vi "LVClass_Image get saturation.vi"(0 "Image in":refnum<class "Image.lvclass">, 7 "Pixels to Average":u32, 11 "error in (no error)":errorcluster) -> (4 "Image out":refnum<class "Image.lvclass">, 10 "Fill Percent":sgl, 15 "error out":errorcluster)   [LabVIEW 2020, in "Image.lvclass"]
doc: "Image statistics computation.\n\n--------------------------------------------------------------------------------\n\n<B>ImageIn </B> : Image object.\n<B>ImageOut </B> : Image object.\n<B>nb_extreme_pixels </B> : Number of pixels to average for min or max computation.\n<B>min </B> : Average of the nb_extreme_pixels greatest elements.\n<B>max </B> : Average of the nb_extreme_pixels smallest elements.\n<B>fill_percentage </B> : Percentage of saturated pixels.\n<B>ErrorIn </B> : Error\n<B>ErrorOut </B> : Error\n\n--------------------------------------------------------------------------------"
uses:
  Image.lvclass
  Image.lvclass/Image.ctl
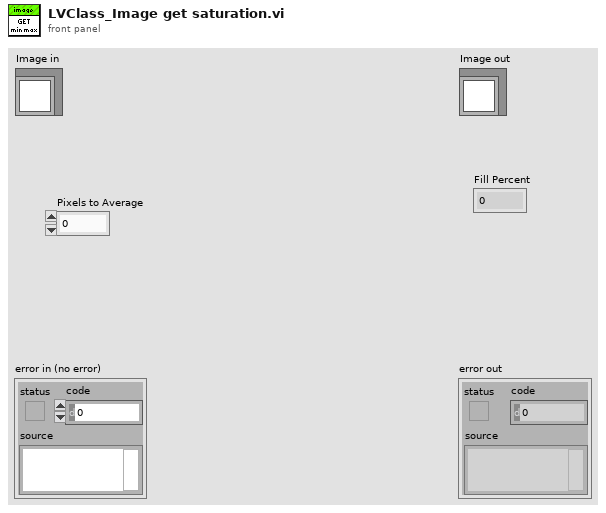
[diagram p1: front panel]
types:
  T1 = typedef "ClassID.ctl" = i64
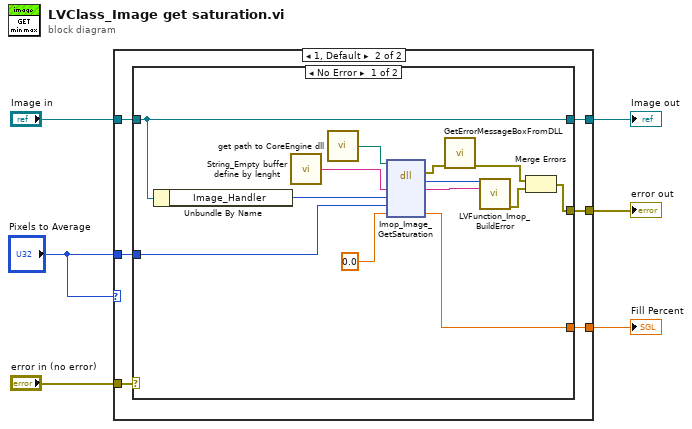
[diagram p0: block diagram]
diagram:
  n1 = case shown="1, Default" "Pixels to Average" {
    tunnel: "error in (no error)" -> [w7 w14]
    tunnel: [w7 w13] -> w5
    tunnel: "Image in" -> [w8 w12]
    tunnel: [w8 w11] -> w3
    tunnel: [_ w10] -> w2
    tunnel: "Pixels to Average" -> [_ w9]
    frame 0 {
    }
    frame 1, Default {
      n2 = case shown="No Error" w14 {
        selector: w14 -> [_ w29]
        tunnel: [w17 w29] -> w13
        tunnel: [w20 w28] -> w11
        tunnel: w12 -> [w20 w28]
        tunnel: [w21 _] -> w10
        tunnel: w9 -> [w15 _]
        frame No Error {
          n3 = Unbundle By Name(w20) -> ("Image_Handler"=w19:T1)
          n4 = call "String_Empty buffer define by lenght.vi"() -> ("Empty buffer"=w27:string)  [unwired: 1 in]
          n5 = call "get path to CoreEngine dll.vi"() -> ("path to wavekit library"=w24:path)  [unwired: 14 in, 1 out]
          n6 = dll-call lib="D:/soft/HASO_v3/SVN_trunk/ImOpCoreEngine4_LV2011/DLLs/c_interface_vc100.dll" fn="Imop_Image_GetSaturation"(path in=w24, "message"=w27, "Image compat"=w19, "Pixels to Average"=w15, "Fill_percent"=sgl 0.0 ("Fill Percent")) -> (error out=w23:errorcluster, "return type"=w26:i32, "message"=w25:string, "Fill_percent"=w21:sgl)  [unwired: 4 in, 1 out]
          n7 = call "GetErrorMessageBoxFromDLL.vi"("error IN"=w23) -> ("error OUT"=w16:errorcluster)  [unwired: 10 in]
          n8 = call "LVFunction_Imop_BuildError.vi"("code"=w26, "String to Prepend to source (\"\")"=w25) -> ("error out"=w18:errorcluster)  [unwired: 13 in]
          n9 = Merge Errors(w16, w18) -> (w17:errorcluster)
        }
        frame Error {
        }
      }
    }
  }
  "error out" <- w5
  "Image out" <- w3
  "Fill Percent" <- w2
